vi "BLM Wait for Move.vi"(0 "PORT Address":refnum<visa-resource-name>, 1 "Motor Address":string="0", 3 "error in (no error)":errorcluster) -> (5 "error out":errorcluster)   [LabVIEW 2016]
panel:
  out "Motor moves":bool
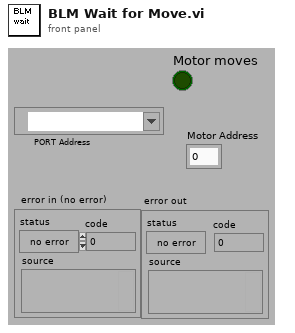
[diagram p1: front panel]
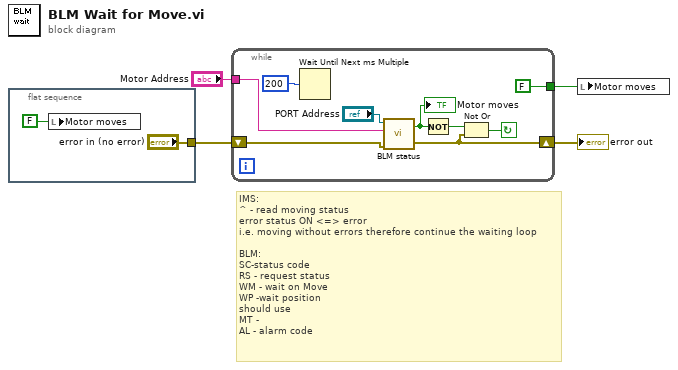
[diagram p0: block diagram]
diagram:
  # "IMS:\n^ - read moving status\nerror status ON <=> error\ni.e. moving without errors therefore continue the waiting loop\n\nBLM:\nSC-status code\nRS - request status\nWM - wait on Move\nWP -wait position\nshould use\nMT - \nAL - alarm code"
  n1 = flat-sequence {
    tunnel: ["error in (no error)"] -> w3
    frame #0 {
      n2 = local write "Motor moves"(FALSE ("Motor moves")) -> ()
    }
  }
  n3 = while {
    shift-left: w3 -> [w12]
    shift-right: [w8] -> w4
    tunnel: "Motor Address" -> [w9]
    tunnel: [FALSE ("Read Echo?")] -> w1
    stop <- w15 continue-if-true
    n4 = Wait Until Next ms Multiple(millisecond multiple=u32 200) -> ()  [unwired: 1 out]
    n5 = call "BLM status.vi"("error in (no error)"=w12, "Motor Address"=w9, "Porty Address"="PORT Address") -> ("error out"=w8:errorcluster, "Motor is moving"=w10:bool)  [unwired: 1 in]
    "Motor moves" <- w10
    n6 = Not(x=w10) -> (.not. x?=w14:bool)
    n7 = Not Or(1:w8, 2:w14) -> (0:w15:bool)
  }
  "error out" <- w4
  n8 = local write "Motor moves"(w1) -> ()
